vi "Set Splash Screen State.vi"(8 "Error In":errorcluster, 11 "Close Splash Screen":bool) -> (0 "Error Out":errorcluster)   [LabVIEW 2014]
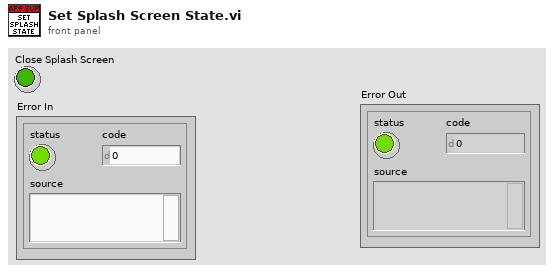
[diagram p1: front panel]
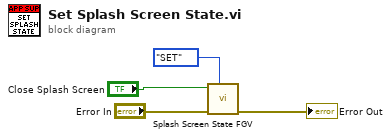
[diagram p0: block diagram]
diagram:
  n1 = call "Splash Screen State FGV.vi"("Operation"=enum16{"GET", "SET"}."SET", "Error In"="Error In", "Close Splash Screen"="Close Splash Screen") -> ("Error Out"=→"Error Out":errorcluster)  [unwired: 7 in, 1 out]
